vi "Write dblEventSignalArray.vi"(8 "error in (no error)":errorcluster, 10 "dblEventSignalArray":T1, 11 "EventPluginBaseClass in":refnum<class "BaseWfrmPlugin.lvclass">) -> (0 "error out":errorcluster, 3 "EventPluginBaseClass out":refnum<class "BaseWfrmPlugin.lvclass">)   [LabVIEW 2014, in "WfrmPlugins.lvlib" / "BaseWfrmPlugin.lvclass"]
uses:
  BaseWfrmPlugin.lvclass
  TypeDefs/dblEvtSignalArray.ctl
  BaseWfrmPlugin.lvclass/BaseWfrmPlugin.ctl
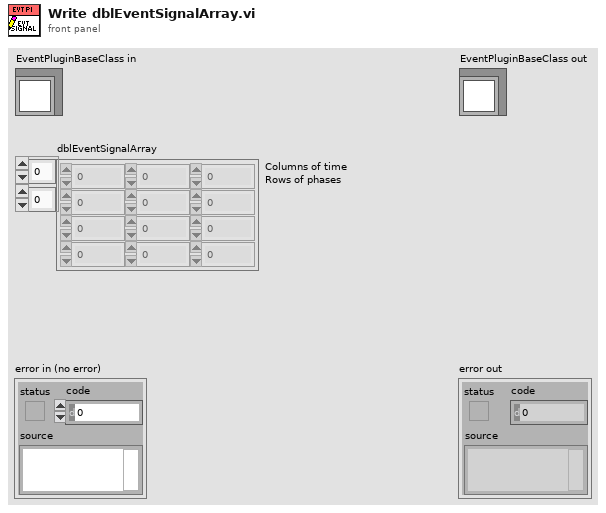
[diagram p1: front panel]
types:
  T1 = typedef "WfrmPlugins.lvlib/BaseWfrmPlugin.lvclass/dblEvtSignalArray.ctl" = dbl[][]
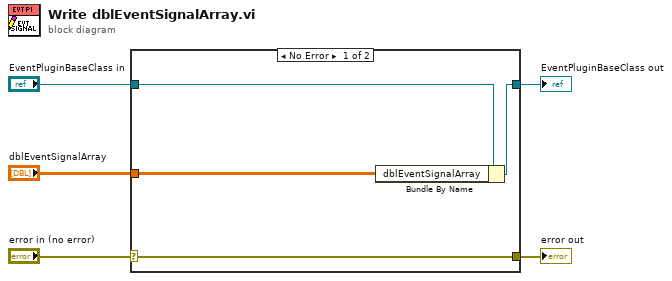
[diagram p0: block diagram]
diagram:
  n1 = case shown="No Error" "error in (no error)" {
    selector: "error in (no error)" -> [w9 w10]
    tunnel: [w9 w10] -> w4
    tunnel: [w7 w11] -> w2
    tunnel: "EventPluginBaseClass in" -> [w8 w11]
    tunnel: "dblEventSignalArray" -> [w6 _]
    frame No Error {
      n2 = Bundle By Name(cluster=w8, "dblEventSignalArray"=w6) -> (w7:refnum<class "BaseWfrmPlugin.lvclass">)
    }
    frame Error {
    }
  }
  "error out" <- w4
  "EventPluginBaseClass out" <- w2
